vi "Startup - Modules Init (SubVI).vi"(8 "Error In":errorcluster, 10 "VIs name":string[](array[string]), 11 "Path to Modules Folder":path) -> (0 "Error Out":errorcluster, 3 "Module Refnum":refnum<vi>[](array[refnum]))   [LabVIEW 2019]
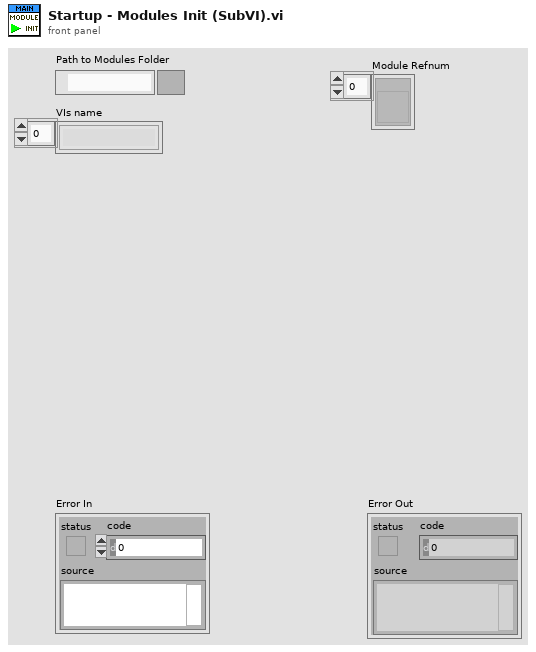
[diagram p1: front panel]
types:
  T1 = enum32{"Bad", "Idle", "Run top level", "Running"}
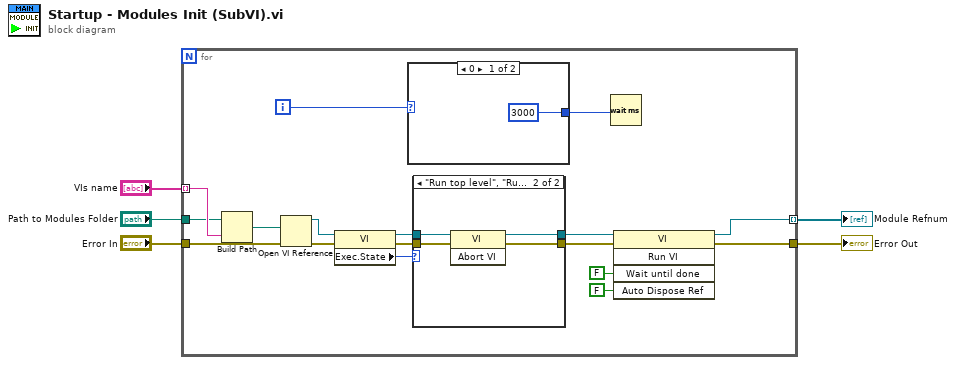
[diagram p0: block diagram]
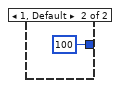
[diagram p2: hidden frame]
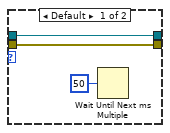
[diagram p3: hidden frame]
diagram:
  n1 = for {
    tunnel: "Error In" -> [w22]
    tunnel: [w21] -> w5
    tunnel: [w20] -> w4 mode=indexing
    tunnel: "VIs name" -> [w17] mode=indexing
    tunnel: "Path to Modules Folder" -> [w16]
    i -> [w7]
    n2 = Build Path(base path=w16, name or relative path=w17) -> (appended path=w15:path)
    n3 = Open VI Reference(vi path=w15, error in (no error)=w22) -> (vi reference=w19:refnum<vi>, error out=w18:errorcluster)  [unwired: 4 in]
    n4 = property class="VI"(reference=w19, error in=w18) -> (reference out=w12:refnum<vi>, error out=w13:errorcluster, "Exec.State"=w14:T1)
    n5 = case shown="0" w7 {
      tunnel: [u32 3000 u32 100] -> w6
      frame 0 {
      }
      frame 1, Default {
      }
    }
    n6 = case shown="\"Run top level\", \"Running\"" w14 {
      tunnel: w13 -> [w26 w31]
      tunnel: w12 -> [w27 w30]
      tunnel: [w27 w29] -> w11
      tunnel: [w26 w28] -> w10
      frame Default {
        n7 = Wait Until Next ms Multiple(millisecond multiple=u32 50) -> ()  [unwired: 1 out]
      }
      frame "Run top level", "Running" {
        n8 = invoke class="VI" method="Abort VI"(reference=w30, error in=w31) -> (reference out=w29:refnum<vi>, error out=w28:errorcluster)  [unwired: 1 in, 1 out]
      }
    }
    n9 = Wait (ms)(milliseconds to wait=w6) -> ()  [unwired: 1 out]
    n10 = invoke class="VI" method="Run VI"(reference=w11, error in=w10, "Wait until done"=FALSE ("Wait Until Done"), "Auto Dispose Ref"=FALSE ("Auto Dispose Reference")) -> (reference out=w20:refnum<vi>, error out=w21:errorcluster)  [unwired: 1 in, 3 out]
  }
  "Error Out" <- w5
  "Module Refnum" <- w4
